vi "Get gRPC ID.vi"(11 "OOP Server in":refnum<class "OCV3.lvclass">) -> (2 "gRPC ID":T1, 3 "OOP Server out":refnum<class "OCV3.lvclass">)   [LabVIEW 2019, in "OCV3.lvlib" / "OCV3.lvclass"]
uses:
  OCV3.lvclass
  gRPC lvSupport/Server API/typeDefs/grpcId.ctl
  OCV3.lvclass/OCV3.ctl
  gRPC lvSupport/gprc-lvsupport.lvlib
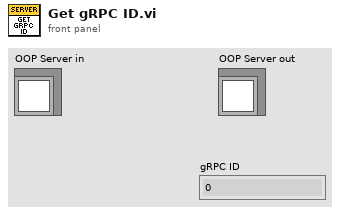
[diagram p1: front panel]
types:
  T1 = typedef "OCV3.lvlib/gprc-lvsupport.lvlib/grpcId.ctl" = u64
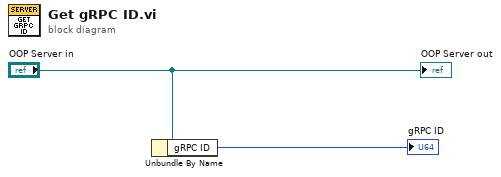
[diagram p0: block diagram]
diagram:
  n1 = Unbundle By Name("OOP Server in") -> ("gRPC ID"=→"gRPC ID":T1)
  "OOP Server out" <- "OOP Server in"
